vi "AcquisitionTimeTracepoint.vi"(7 "service name":string, 8 "error in (no error)":errorcluster, 10 "acq time":u32, 11 "Qbus in":refnum<class "Qbus.lvclass">) -> (0 "error out":errorcluster)   [LabVIEW 2017]
uses:
  <vilib>/addons/Qbus/Qbus.lvclass
  <vilib>/addons/TraceLogger/TraceLogger.lvlib
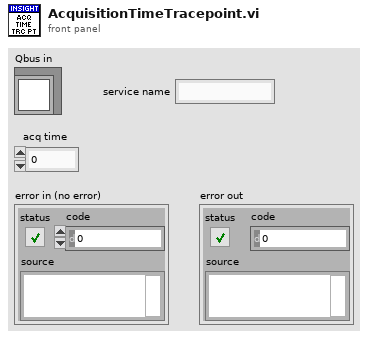
[diagram p1: front panel]
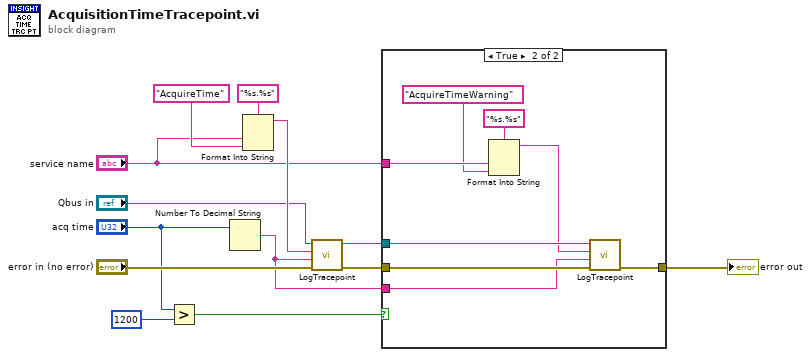
[diagram p0: block diagram]
diagram:
  n1 = Greater?(x="acq time", y=u32 1200) -> (0:w7:bool)
  n2 = Number To Decimal String(number="acq time") -> (decimal integer string=w1:string)  [unwired: 1 in]
  n3 = Format Into String(format string="%s.%s", "service name", "AcquireTime" ("tracepoint")) -> (resulting string=w8:string)  [unwired: 2 in, 1 out]
  n4 = call <vilib>:"LogTracepoint.vi"("error in (no error)"="error in (no error)", "log string"=w1, "tracepoint"=w8, "qbus in"="Qbus in") -> ("error out"=w5:errorcluster, "qbus out"=w2:refnum<class "Qbus.lvclass">)  [unwired: 6 in]
  n5 = case shown="True" w7 {
    tunnel: [w14 w21] -> w6
    tunnel: w5 -> [w14 w22]
    tunnel: "service name" -> [_ w19]
    tunnel: w2 -> [_ w17]
    tunnel: w1 -> [_ w15]
    frame False {
    }
    frame True {
      n6 = Format Into String(format string="%s.%s", w19, "AcquireTimeWarning" ("tracepoint")) -> (resulting string=w16:string)  [unwired: 2 in, 1 out]
      n7 = call <vilib>:"LogTracepoint.vi"("error in (no error)"=w22, "log string"=w15, "tracepoint"=w16, "qbus in"=w17) -> ("error out"=w21:errorcluster)  [unwired: 6 in, 1 out]
    }
  }
  "error out" <- w6
